vi "Practica 4.vi"() -> ()   [LabVIEW 2014]
uses:
  Practica 4.ctl
  <vilib>/LabVIEW Interface for Arduino/Type Defs/Board Type.ctl
  <vilib>/LabVIEW Interface for Arduino/Type Defs/Pin Mode.ctl
  Global personas.vi
  <vilib>/LabVIEW Interface for Arduino/LabVIEW Interface for Arduino.lvlib
panel:
  in  "Nivel de Luz":u8(slide) scale=0.0..100.0
  in  "Temperatura Maxima":dbl
  out "Temperatura":dbl(slide) scale=0.0..100.0
  in  "Board Type":T1
  in  "VISA resource":refnum<visa-resource-name>
  out "?":T2
  out "Personas":dbl
  out "Información":string
  in  "Parar":bool
  in  "Capacidad Maxima":dbl
  # "Temperatura"
  # "Iluminación"
  # "Ingreso"
  # "Control"
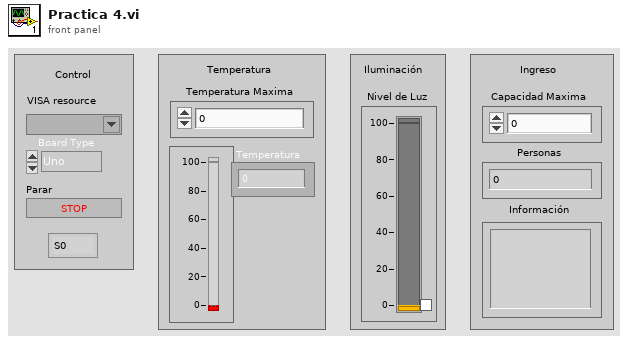
[diagram p1: front panel]
types:
  T1 = typedef "LabVIEW Interface for Arduino.lvlib/Board Type.ctl" = enum16{"Uno", "Dimuelanove w/Atmega 328", "Mega 2560"}
  T2 = typedef "Practica 4.ctl" = enum16{"S0", "S1", "S2", "S3", "S4"}
  T3 = typedef "LabVIEW Interface for Arduino.lvlib/Arduino Resource.ctl" = cluster{"VISA resource":refnum<visa-resource-name>, "Board Type":T1, "Connection Type":enum8{"USB / Serial"}, "Bytes Per Packet (15)":u8}
  T4 = enum8{"Enabled", "Disabled", "Disabled and Grayed Out"}
  T5 = typedef "LabVIEW Interface for Arduino.lvlib/Pin Mode.ctl" = enum8{"Input", "Output"}
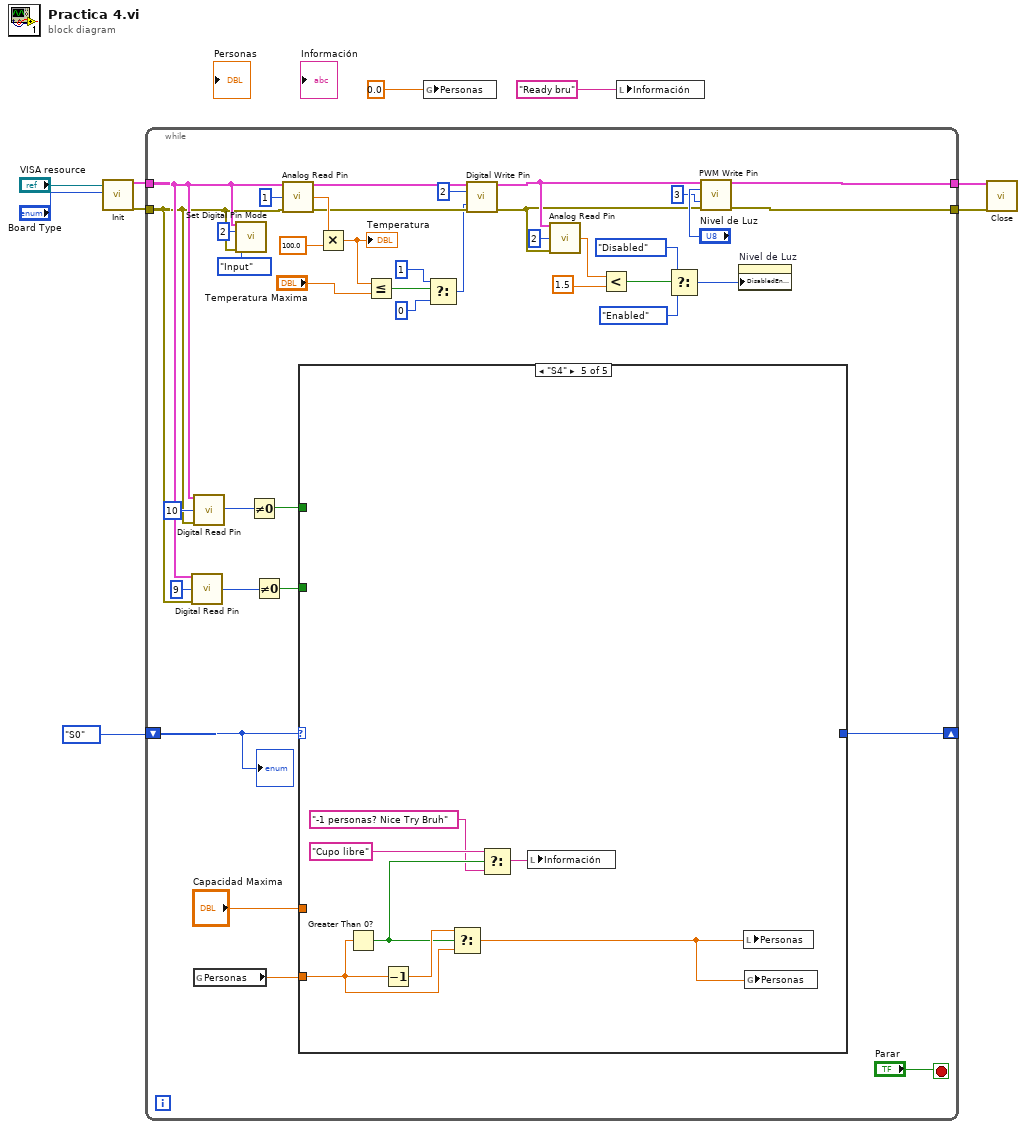
[diagram p0: block diagram]
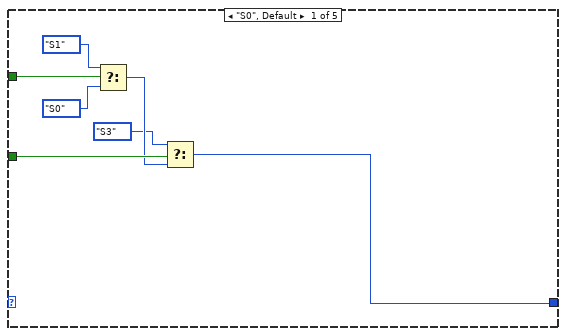
[diagram p2: hidden frame]
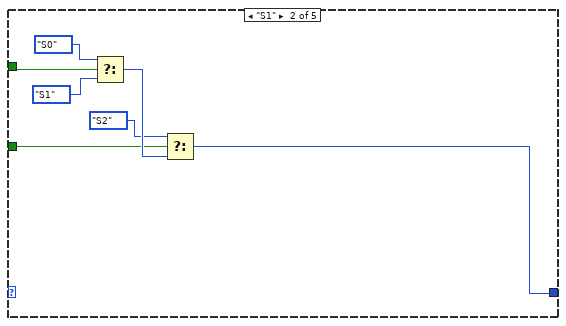
[diagram p3: hidden frame]
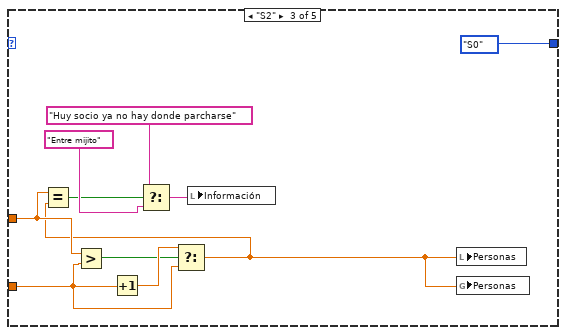
[diagram p4: hidden frame]
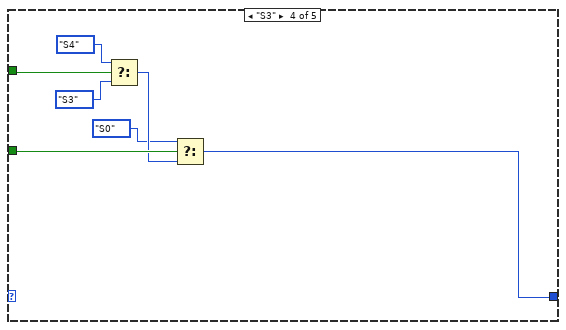
[diagram p5: hidden frame]
diagram:
  n1 = call <vilib>:"Init.vi"("VISA resource"="VISA resource", "Board Type (Uno)"="Board Type") -> ("Arduino Resource"=w3:T3, "error out"=w2:errorcluster)  [unwired: 16 in]
  n2 = while {
    shift-right: [w47] -> _
    shift-left: Practica_4."S0" -> [w45]
    tunnel: [w33] -> w4
    tunnel: w3 -> [w23]
    tunnel: w2 -> [w22]
    tunnel: [w32] -> w1
    stop <- "Parar" stop-if-true
    n3 = call <vilib>:"Digital Read Pin.vi"("Arduino Resource"=w23, "Digital I/O Pin (0)"=u8 9, "error in"=w22) -> ("Value"=w27:u8)  [unwired: 10 in, 2 out]
    n4 = call <vilib>:"Digital Read Pin.vi"("Arduino Resource"=w23, "Digital I/O Pin (0)"=u8 10, "error in"=w22) -> ("Value"=w29:u8)  [unwired: 10 in, 2 out]
    n5 = global read "Global personas.vi" "Personas"() -> (w46:dbl)
    n6 = call <vilib>:"Set Digital Pin Mode.vi"("Arduino Resource"=w23, "Digital I/O Pin"=u8 2, "Pin Mode (Input)"=Pin_Mode."Input", "error in"=w22) -> ()  [unwired: 10 in, 2 out]
    n7 = Not Equal To 0?(x=w29) -> (x != 0?=w28:bool)
    n8 = Not Equal To 0?(x=w27) -> (x != 0?=w26:bool)
    n9 = call <vilib>:"Analog Read Pin.vi"("Arduino Resource"=w23, "Analog Input Pin (0)"=u8 1, "error in"=w22) -> ("Arduino Resource"=w38:T3, "Voltage"=w43:dbl, "error out"=w37:errorcluster)  [unwired: 10 in]
    n10 = case shown="\"S4\"" w45 {
      tunnel: w28 -> [w56 w63 _ w80 _]
      tunnel: w26 -> [w53 w58 _ w77 _]
      tunnel: "Capacidad Maxima" -> [_ _ w66 _ _]
      tunnel: [w50 w57 Practica_4."S0" w74 _] -> w47
      tunnel: w46 -> [_ _ w65 _ w86]
      frame "S0", Default {
        n11 = Select(t=Practica_4."S1", s=w56, f=Practica_4."S0") -> (s? t:f=w52:T2)
        n12 = Select(t=Practica_4."S3", s=w53, f=w52) -> (s? t:f=w50:T2)
      }
      frame "S1" {
        n13 = Select(t=Practica_4."S0", s=w63, f=Practica_4."S1") -> (s? t:f=w60:T2)
        n14 = Select(t=Practica_4."S2", s=w58, f=w60) -> (s? t:f=w57:T2)
      }
      frame "S2" {
        n15 = Greater?(x=w66, y=w65) -> (0:w72:bool)
        n16 = Increment(x=w65) -> (x+1=w73:dbl)
        n17 = Select(t=w73, s=w72, f=w65) -> (s? t:f=w64:dbl)
        n18 = Equal?(x=w66, y=w64) -> (x = y?=w67:bool)
        n19 = Select(t="Huy socio ya no hay donde parcharse", s=w67, f="Entre mijito") -> (s? t:f=w68:string)
        n20 = local write "Información"(w68) -> ()
        n21 = local write "Personas"(w64) -> ()
        n22 = global write "Global personas.vi" "Personas"(w64) -> ()
      }
      frame "S3" {
        n23 = Select(t=Practica_4."S4", s=w80, f=Practica_4."S3") -> (s? t:f=w76:T2)
        n24 = Select(t=Practica_4."S0", s=w77, f=w76) -> (s? t:f=w74:T2)
      }
      frame "S4" {
        n25 = Greater Than 0?(x=w86) -> (x > 0?=w85:bool)
        n26 = Decrement(x=w86) -> (x-1=w87:dbl)
        n27 = Select(t=w87, s=w85, f=w86) -> (s? t:f=w81:dbl)
        n28 = Select(t="Cupo libre", s=w85, f="-1 personas? Nice Try Bruh") -> (s? t:f=w82:string)
        n29 = local write "Información"(w82) -> ()
        n30 = local write "Personas"(w81) -> ()
        n31 = global write "Global personas.vi" "Personas"(w81) -> ()
      }
    }
    n32 = Multiply(x=w43, y=100.0) -> (x*y=w40:dbl)
    "Temperatura" <- w40
    n33 = Less Or Equal?(x=w40, y="Temperatura Maxima") -> (x <= y?=w39:bool)
    n34 = Select(t=u8 1 ("Value (0)"), s=w39, f=u8 0 ("Value (0)")) -> (s? t:f=w35:u8)
    n35 = call <vilib>:"Digital Write Pin.vi"("Arduino Resource"=w38, "Digital I/O Pin (0)"=u8 2, "Value (0)"=w35, "error in"=w37) -> ("Arduino Resource"=w18:T3, "error out"=w17:errorcluster)  [unwired: 10 in]
    n36 = call <vilib>:"Analog Read Pin.vi"("Arduino Resource"=w18, "Analog Input Pin (0)"=u8 2, "error in"=w17) -> ("Voltage"=w15:dbl)  [unwired: 10 in, 2 out]
    n37 = Less?(x=w15, y=1.5) -> (x < y?=w13:bool)
    n38 = Select(t=T4."Disabled" ("Disabled"), s=w13, f=T4."Enabled" ("Disabled")) -> (s? t:f=w12:T4)
    n39 = call <vilib>:"PWM Write Pin.vi"("Arduino Resource"=w18, "Duty Cycle (0 - 255)"="Nivel de Luz", "PWM Pin (3)"=u8 3 ("Analog Input Pin (0)"), "error in"=w17) -> ("Arduino Resource"=w33:T3, "error out"=w32:errorcluster)  [unwired: 10 in]
    n40 = property on="Nivel de Luz" class="Slide (strict)"("DisabledEnum"=w12) -> ()  [unwired: 2 in, 2 out]
    "?" <- w45
  }
  n41 = global write "Global personas.vi" "Personas"(0.0 ("Personas")) -> ()
  n42 = local write "Información"("Ready bru") -> ()
  n43 = call <vilib>:"Close.vi"("Arduino Resource"=w4, "error in"=w1) -> ()  [unwired: 13 in, 1 out]
